vi "Get is running.vi"(8 "error in (no error)":errorcluster, 11 "AOTF in":refnum<class "AOTF.lvclass">) -> (0 "error out":errorcluster, 2 "is running?":bool, 3 "AOTF out":refnum<class "AOTF.lvclass">)   [LabVIEW 2012, in "AOTF.lvclass"]
uses:
  AOTF.lvclass
  AOTF.lvclass/AOTF.ctl
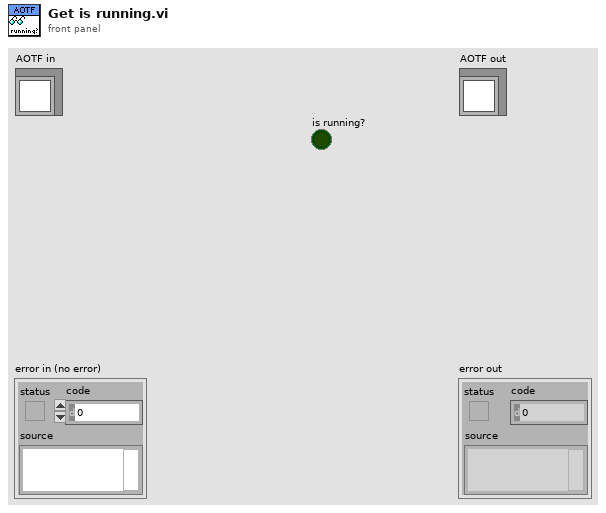
[diagram p1: front panel]
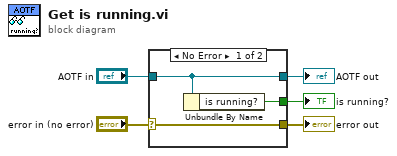
[diagram p0: block diagram]
diagram:
  n1 = case shown="No Error" "error in (no error)" {
    selector: "error in (no error)" -> [w8 w10]
    tunnel: [w8 w10] -> w4
    tunnel: [w7 w9] -> w2
    tunnel: "AOTF in" -> [w7 w9]
    tunnel: [w6 _] -> w1
    frame No Error {
      n2 = Unbundle By Name(w7) -> ("is running?"=w6:bool)
    }
    frame Error {
    }
  }
  "error out" <- w4
  "AOTF out" <- w2
  "is running?" <- w1
